vi "UniCyRO_Sim.vi"() -> ()   [LabVIEW 2012]
doc: "This VI starts and stops the environment simulator and serves as the master VI for your simulation code. Open and run this VI to display the environment simulator, or open the block diagram to view or modify simulation code."
uses:
  <vilib>/Simulation/Scripting/Companion Diagram/SimConfigNode/SimParams.ctl
  <vilib>/Simulation/Scripting/Companion Diagram/SimConfigNode/_simSolvers.ctl
  <vilib>/Simulation/Implementation/Shared/SIMSCR Execution Mode.ctl
  <vilib>/Simulation/Param Hierarchy/Typedefs/SIMPH Param Control Actions.ctl
  <vilib>/Simulation/Implementation/Shared/NILVSim_ParamChanged.vi
  <vilib>/Simulation/Implementation/Shared/NILVSim_Manager.vi
  <vilib>/Simulation/Implementation/Shared/NILVSim_FinalizeModel.vi
  <vilib>/Simulation/Implementation/Shared/SIM Unbundle Sim Info.vi
  <vilib>/Utility/error.llb/Clear Errors.vi
  <vilib>/Simulation/Implementation/Shared/NILVSim_GetModelError.vi
  <vilib>/Simulation/Implementation/Shared/SIM Bundle Sim Info.vi
  <vilib>/Simulation/Implementation/Shared/NILVSim_Initialize.vi
  <vilib>/Simulation/Utility/Implementation/NILVSim Get Time and IsAcceptedStep.vi
  <vilib>/Simulation/Implementation/Shared/SIMSH Read Queue.vi
  Model/UniCyRO/UniCyRO_Host_Sim.lvclass
  <vilib>/Simulation/Implementation/XNodeFramework/SimXNode/SimX.xnode
  <vilib>/Simulation/Model Libraries/PID/SIM PID (Academic).vi
  <vilib>/Simulation/Model Libraries/PID/SIM PID.vi
  <vilib>/Simulation/Scripting/Companion Diagram/SimConfigNode/SimDog.xnode
  <vilib>/robotics/Simulator/NI_Robotics_Simulator.lvlib
  <vilib>/Simulation/Implementation/Shared/NI_SIM_Implementation.lvlib
panel:
  in  "Derivative time [s] (Td)":dbl=1.0
  in  "Integral time [s] (Ti)":dbl=1.0
  in  "Proportional Gain (Kc)":dbl=1.0
  in  "Gain":dbl(slide) scale=-100.0..100.0
  out "Waveform Chart":cluster{"Accel_Y (g)":dbl}(graph)
  in  "stop":bool
  in  "3D Visualization":refnum<vi>(3d-picture)
  in  "Gyro Motor ccw velocity (rad/s)":dbl(slide) scale=-100.0..100.0
  out "Drive Motor ccw velocity (rad/s)":dbl(slide) scale=-100.0..100.0
  in  "Torsion Motor ccw velocity (rad/s)":dbl(slide) scale=-1000.0..1000.0
  in  "manifest filename":string="UniCyRO_Sim.xml"
  # "Instructions:\n\n1. Run this VI.  \n\n2. The robot balances upright"
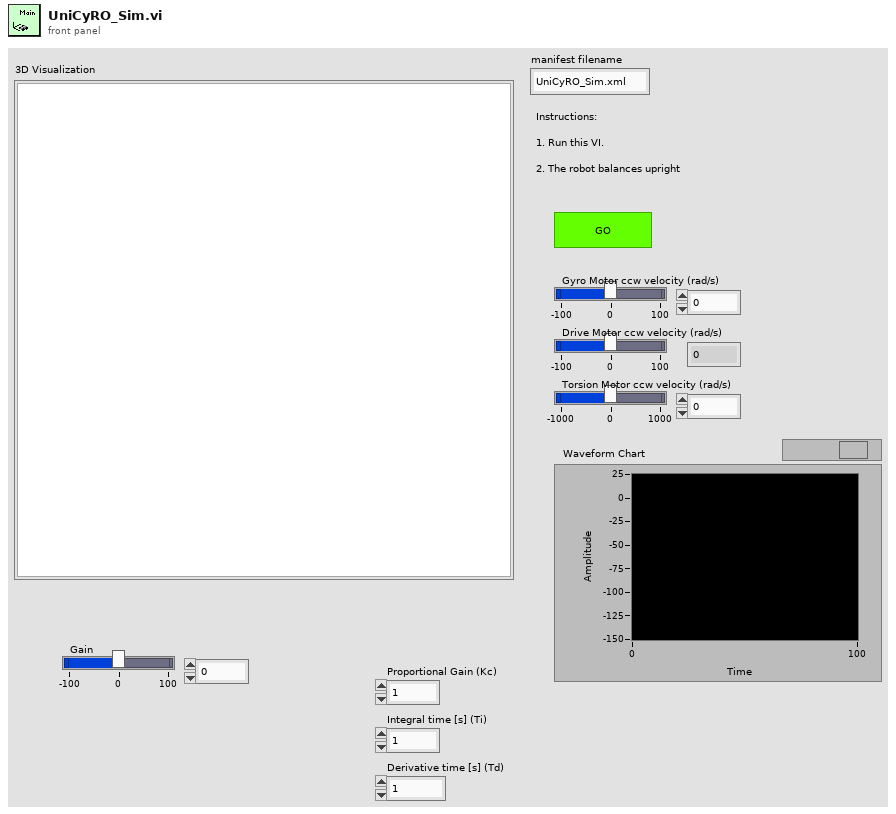
[diagram p1: front panel]
types:
  T1 = enum16{"Simulate to Completion", "Single Time-Step Simulation (Fixed Step Only)"}
  T2 = typedef "SIMSCR Execution Mode.ctl" = enum16{"Simulate to Completion", "Single Time-Step Simulation (Fixed Step Only)"}
  T3 = typedef "SIMPH Param Control Actions.ctl" = enum16{"get params", "set params"}
  T4 = cluster{"SIMSH Sim Time":dbl, "SIM PID Derivative Gain.vi":cluster{"output":dbl}, "SIM PID Derivative Gain.vi - SIMSH":cluster{"SIMSH Sim Time":dbl, "t 3":dbl, "Select 2":cluster{"s? t:f":dbl}, "Equal?":cluster{"x = y?":bool}, "Or":cluster{"x .or. y?":bool}, "Equal To 0?":cluster{"x = 0?":bool}}, "High Frequency [s] (Tf)":dbl, "Gain":cluster{"output":dbl}, "Summation":cluster{"Result":dbl}, "Integral Gain - series.vi":cluster{"output":dbl}, "Integral Gain - series.vi - SIMSH":cluster{"SIMSH Sim Time":dbl, "Select 2":cluster{"s? t:f":dbl}, "integral in gain?":bool, "Integrator":cluster{"output y(k)":dbl}, "Gain 2":cluster{"output":dbl}, "Select":cluster{"s? t:f":dbl}, "Equal To 0?":cluster{"x = 0?":bool}, "Reciprocal":cluster{"1/x":dbl}}}
  T5 = typedef "SimParams.ctl" = cluster{"Initial Time (s)":dbl, "Final Time (s)":dbl, "Step Size (s)":dbl, "ODE Solver":T6, "Minimum Step Size (s)":dbl, "Maximum Step Size (s)":dbl, "Relative Tolerance":dbl, "Absolute Tolerance":dbl, "Software Timing":bool, "Initial Step Size (s)":dbl, "Automatic Fixed Step Size?":bool, "Automatic Discrete Step Size?":bool, "Discrete Step Size (s)":dbl, "Calculate using Time Step":bool, "Solver Wired?":bool, "Prev.Frm.Expected End":u64, "Prev.Frm.Actual End":u64, "Prev.Frm.Finished Late?":bool, "Prev.Iter.Expected End":u64, "Prev.Iter.Actual End":u64, "Prev.Iter.Finished Late?":bool, "Expected Iteration Start":u64, "Actual Iteration Start":u64, "Expected Frame Start":u64, "Actual Frame Start":u64, "Source Name":string, "Name":string, "Period":i64, "Deadline":i64, "Offset":i64, "Start":i64, "Priority":i32, "Timeout":i32, "Processor":i32, "Mode":enum32{"No Change", "Process missed periods, maintain original phase", "Discard missed periods, maintain original phase", "Process missed periods, ignore original phase", "Discard missed periods, ignore original phase"}, "Wakeup reason":enum32{"Normal", "Aborted", "Asynchronous wakeup", "Timing source error", "Timed loop error", "Timeout"}, "Error":errorcluster, "Source Type":string, "Secondary Source Type":string, "Global End Time":u64, "Global Start Time":u64, "Full Solver Reset":bool, "Execution Mode":T2, "Nan/Inf Check":bool, "Custom Solver Library":string, "Solver Is Variable":bool, "custom solver name":string, "Signal Collection Decimation":u32}
  T6 = typedef "_simSolvers.ctl" = enum16{"Runge-Kutta 1 (Euler)", "Runge-Kutta 2", "Runge-Kutta 3", "Runge-Kutta 4", "Runge-Kutta 23 (variable)", "Runge-Kutta 45 (variable)", "BDF (variable)", "Adams-Moulton (variable)", "Rosenbrock (variable)", "Discrete States Only", "SDIRK 4 (variable)", "Radau 5 (variable)", "Radau 9 (variable)", "Radau 13 (variable)", "Radau [Variable Order] (variable)", "Gear's Method (variable)", "Linearizer", "State Query", "Trim Eval", "Custom Solver"}
  T7 = cluster{"IMU Data":cluster{"Accelerometer Data":cluster{"Accel_X (g)":dbl, "Accel_Y (g)":dbl, "Accel_Z (g)":dbl}, "Gyros Data":cluster{"Pitch (deg/s)":dbl, "Roll (deg/s)":dbl, "Yaw (deg/s)":dbl}}, "LIDAR Data":cluster{"Magnitude":dbl[], "Direction":dbl[]}, "GPS Data":cluster{"Latitude (degree)":dbl, "Longitude (degree)":dbl, "Time Stamp":timestamp, "Speed Over Ground (knots)":dbl, "Bearing (degree)":dbl}, "Compass Data":cluster{"Acceleration":cluster{"x (g)":dbl, "y (g)":dbl, "z (g)":dbl}, "Magnetic Field":cluster{"x (gauss)":dbl, "y (gauss)":dbl, "z (gauss)":dbl}, "Heading Data":cluster{"Head (deg)":dbl, "Pitch (deg)":dbl, "Roll (deg)":dbl}, "Tilt Data":cluster{"Pitch (deg)":dbl, "Roll (deg)":dbl, "Temperature (deg)":dbl}}}
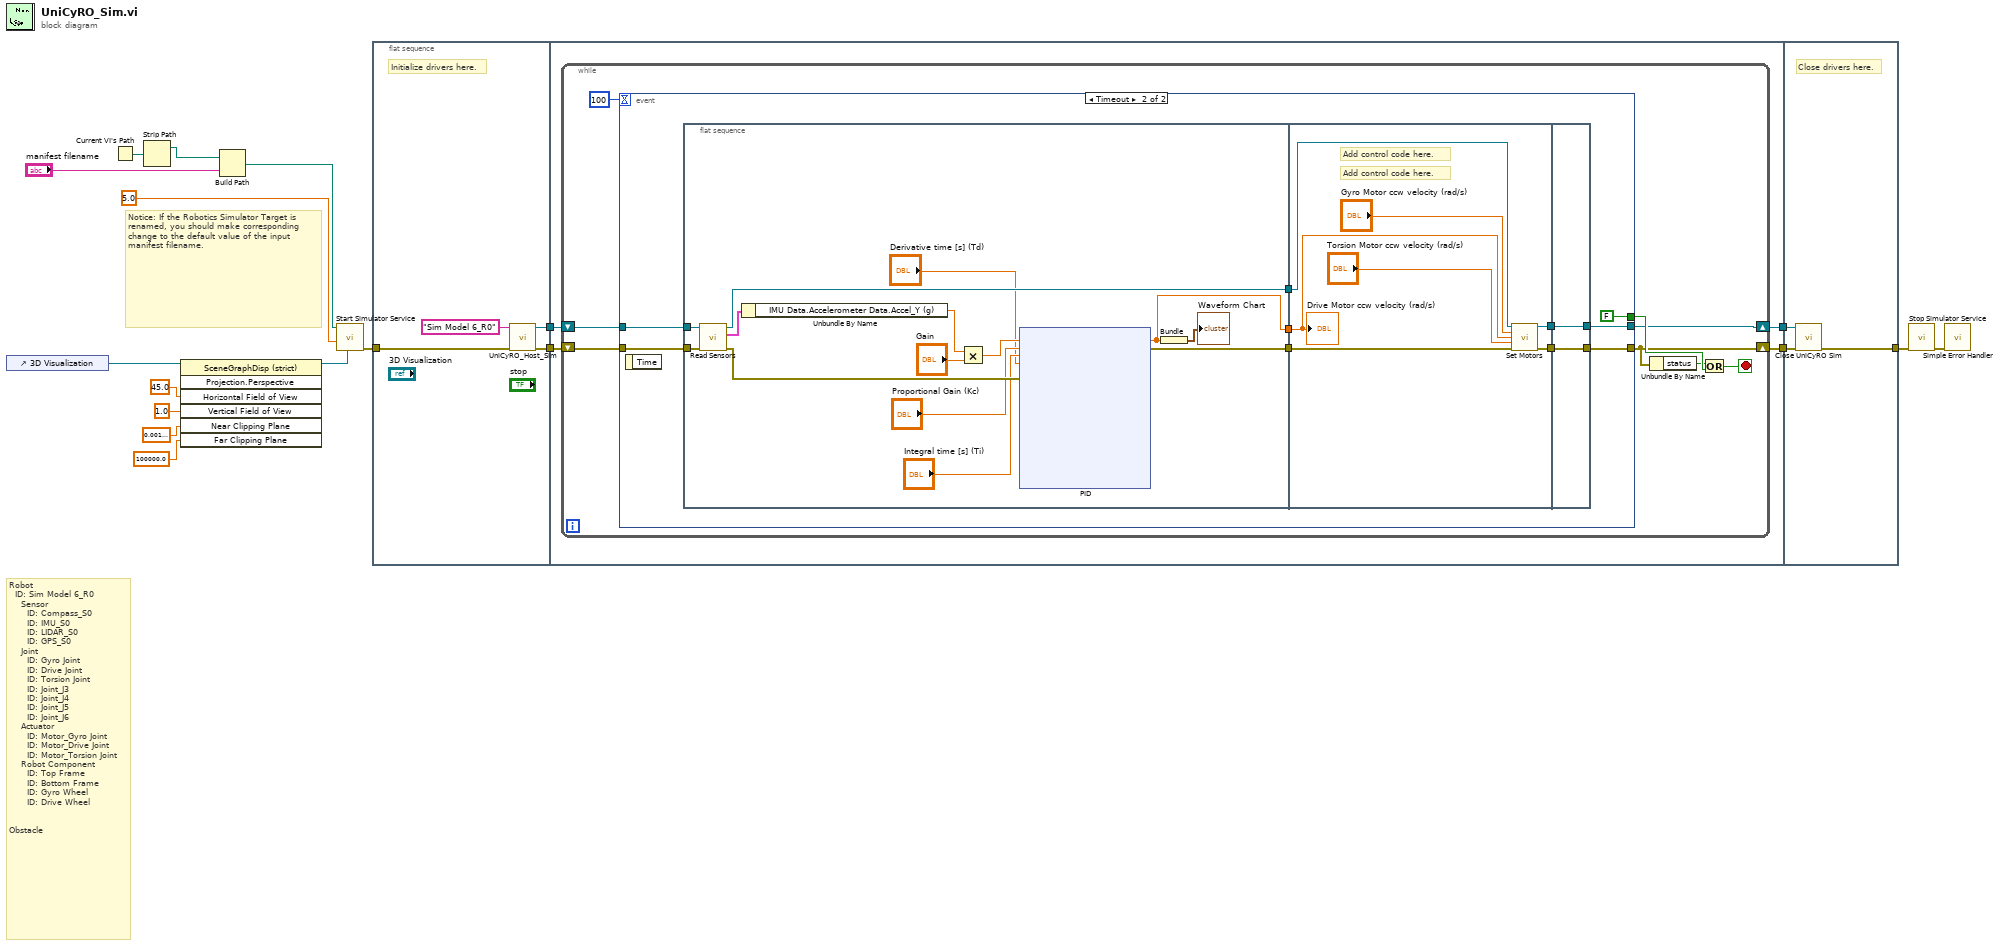
[diagram p0: block diagram]
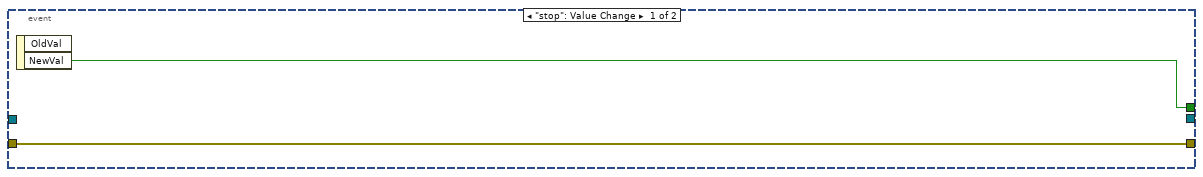
[diagram p2: hidden frame]
diagram:
  # "Robot\n\t\tID: Sim Model 6_R0\n\t\t\t\tSensor\n\t\t\t\t\t\tID: Compass_S0\n\t\t\t\t\t\tID: IMU_S0\n\t\t\t\t\t\tID: LIDAR_S0\n\t\t\t\t\t\tID: GPS_S0\n\t\t\t\tJoint\n\t\t\t\t\t\tID: Gyro Joint\n\t\t\t\t\t\tID: Drive Joint\n\t\t\t\t\t\tID: Torsion Joint\n\t\t\t\t\t\tID: Joint_J3\n\t\t\t\t\t\tID: Joint_J4\n\t\t\t\t\t\tID: Joint_J5\n\t\t\t\t\t\tID: Joint_J6\n\t\t\t\tActuator\n\t\t\t\t\t\tID: Motor_Gyro Joint\n\t\t\t\t\t\tID: Motor_Drive Joint\n\t\t\t\t\t\tID: Motor_Torsion Joint\n\t\t\t\tRobot Component\n\t\t\t\t\t\tID: Top Frame\n\t\t\t\t\t\tID: Bottom Frame\n\t\t\t\t\t\tID: Gyro Wheel\n\t\t\t\t\t\tID: Drive Wheel\n\n\nObstacle"
  # "Notice: If the Robotics Simulator Target is renamed, you should make corresponding change to the default value of the input manifest filename."
  n1 = control-ref of="3D Visualization"() -> (w2:refnum<vi>)
  n2 = Current VI's Path() -> (path=w16:path)
  n3 = Strip Path(path=w16) -> (stripped path=w15:path)  [unwired: 1 out]
  n4 = invoke on="Invoke Node" class="SceneGraphDisp (strict)" method="Projection.Perspective"(reference=w2, "Horizontal Field of View"=sgl 45.0 ("Field of View"), "Vertical Field of View"=sgl 1.0 ("Aspect Ratio"), "Near Clipping Plane"=sgl 0.001, "Far Clipping Plane"=sgl 100000.0) -> (reference out=w1:refnum<vi>)  [unwired: 2 in, 6 out]
  n5 = Build Path(base path=w15, name or relative path="manifest filename") -> (appended path=w14:path)
  n6 = call <vilib>:"Start Simulator Service.vi"("3D picture refnum"=w1, "step size (ms)"=5.0 ("stepsize(ms)"), "manifest file"=w14) -> ("error out"=w11:errorcluster)  [unwired: 8 in]
  n7 = flat-sequence {
    tunnel: w11 -> [w22]
    tunnel: [w21] -> w10
    tunnel: [w19] -> w8
    tunnel: w10 -> [w25]
    tunnel: [w26] -> w9
    tunnel: w8 -> [w24]
    tunnel: [w23] -> w7
    tunnel: [w309] -> w17
    tunnel: w9 -> [w310]
    tunnel: w7 -> [w311]
    frame #0 {
      # "Initialize drivers here."
      n8 = call "UniCyRO_Host_Sim"("error in (no error)"=w22, "robot ID"="Sim Model 6_R0") -> ("error out"=w21:errorcluster, "UniCyRO_Host_Sim out"=w19:refnum<class "UniCyRO_Host_Sim.lvclass">)  [unwired: 8 in]
    }
    frame #1 {
      n9 = while {
        shift-right: [w30] -> w26
        shift-left: w25 -> [w33]
        shift-right: [w27] -> w23
        shift-left: w24 -> [w28]
        stop <- w31 stop-if-true
        n10 = event shown="[1] Timeout" {
          selector: _ -> [_ _]
          dyn-events: _ -> [_ _]
          timeout: 100 -> [_ _]
          tunnel: [w35 FALSE ("stop")] -> w32
          tunnel: [w36 w44] -> w30
          tunnel: w33 -> [w36 w45]
          tunnel: w28 -> [_ w43]
          tunnel: [_ w42] -> w27
          event "stop": Value Change {
            n11 = event-data() -> ("NewVal"=w35:bool)  [unwired: 1 in, 1 out]
          }
          event Timeout {
            n12 = event-data() -> ()  [unwired: 1 in, 1 out]
            n13 = flat-sequence {
              tunnel: w43 -> [w60]
              tunnel: w45 -> [w59]
              tunnel: [w58] -> w39
              tunnel: [w53] -> w38
              tunnel: [w54] -> w37
              tunnel: [w303] -> w41
              tunnel: [w301] -> w40
              tunnel: w39 -> [w302]
              tunnel: w38 -> [w300]
              tunnel: w37 -> [w304]
              tunnel: [w308] -> w42
              tunnel: [w307] -> w44
              tunnel: w41 -> [w307]
              tunnel: w40 -> [w308]
              frame #0 {
                n14 = call "Read Sensors.vi"("error in (no error)"=w59, "UniCyRO_Host_Sim in"=w60) -> ("error out"=w55:errorcluster, "Data"=w57:T7, "UniCyRO_Host_Sim out"=w58:refnum<class "UniCyRO_Host_Sim.lvclass">)  [unwired: 5 in]
                n15 = Unbundle By Name(w57) -> ("IMU Data.Accelerometer Data.Accel_Y (g)"=w52:dbl)
                n16 = Multiply(x=w52, y="Gain") -> (x*y=w51:dbl)
                n17 = xnode "PID"("Error"=w51, "Proportional Gain (Kc)"="Proportional Gain (Kc)", "Integral time [s] (Ti)"="Integral time [s] (Ti)", "Derivative time [s] (Td)"="Derivative time [s] (Td)", "error in"=w55) -> ("Output"=w53:dbl, "error out"=w54:errorcluster)  [unwired: 1 in, 10 out]
                n18 = Bundle("Output"=w53) -> (→"Waveform Chart":cluster{"Output":dbl})  [unwired: 1 in]
              }
              frame #1 {
                # "Add control code here."
                # "Add control code here."
                n19 = call "Set Motors.vi"("UniCyRO_Host_Sim in"=w302, "Gyro Motor ccw velocity (rad/s)"="Gyro Motor ccw velocity (rad/s)", "Drive Motor ccw velocity (rad/s)"=w300, "Torsion Motor ccw velocity (rad/s)"="Torsion Motor ccw velocity (rad/s)", "error in (no error)"=w304) -> ("UniCyRO_Host_Sim out"=w301:refnum<class "UniCyRO_Host_Sim.lvclass">, "error out"=w303:errorcluster)  [unwired: 9 in]
                "Drive Motor ccw velocity (rad/s)" <- w300
              }
              frame #2 {
              }
            }
          }
        }
        n20 = Unbundle By Name(w30) -> ("status"=w29:bool)
        n21 = Or(x=w29, y=w32) -> (x .or. y?=w31:bool)
      }
    }
    frame #2 {
      # "Close drivers here."
      n22 = call "Close UniCyRO Sim.vi"("error in (no error)"=w310, "UniCyRO_Host_Sim in"=w311) -> ("error out"=w309:errorcluster)  [unwired: 9 in]
    }
  }
  n23 = call <vilib>:"Stop Simulator Service.vi"("error in (no error)"=w17) -> ("error out"=w12:errorcluster)  [unwired: 10 in]
  n24 = call <vilib>:"Simple Error Handler.vi"("error in (no error)"=w12) -> ()  [unwired: 4 in, 5 out]
